vi "CSMP-PostPostMsg.vi"(0 "state":string, 1 "args":string, 2 "source/target":string, 3 "Pre-State in":string, 4 "Pre-Args in":string, 5 "Error in":errorcluster caption="Error in (no error)", 6 "session error":errorcluster, 8 "Module Name":string, 10 "Response Arguments":string) -> (14 "state out":string, 15 "args out":string, 16 "source/target out":string, 17 "Pre-State out":string, 18 "Pre-Args out":string, 19 "error":errorcluster)   [LabVIEW 2020, in "Communicable State Machine.lvlib"]
uses:
  Communicable State Machine.lvlib
  _CSM_MSG_TYPE.ctl
  _Cross CSM State Data.ctl
  _Cross CSM State Response.ctl
  _CSM_Response Source Message.ctl
  Priority Queue.lvclass/Priority Queue.ctl
  Enqueue Element.vi
  _CSMOFGV.vi
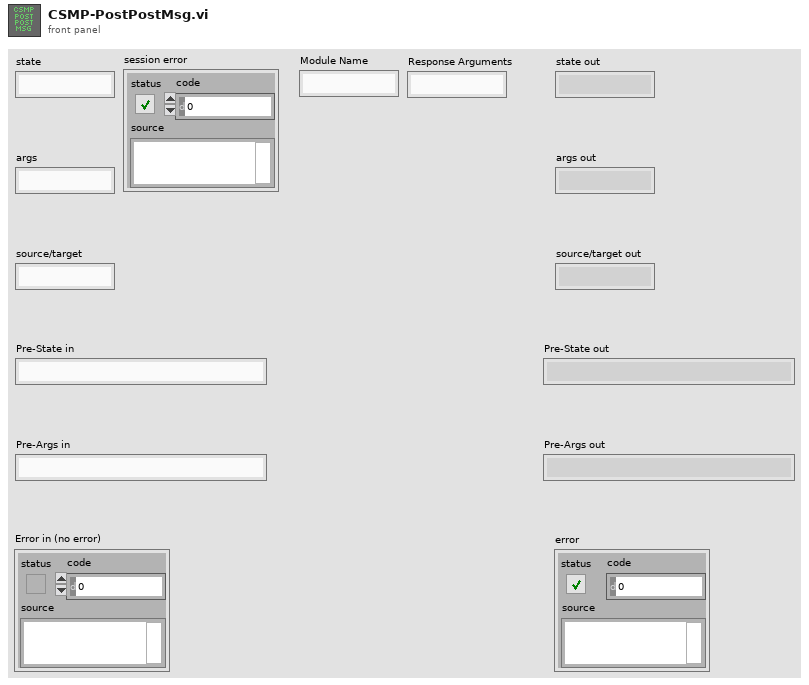
[diagram p1: front panel]
types:
  T1 = typedef "Communicable State Machine.lvlib/_CSMObj.ctl" = cluster{"Requested Name":string, "Module Name":string, "Mode":T2, "Queue":refnum<class "Priority Queue.lvclass">, "CSM-Data":refnum<data-value>, "User Event":refnum<user-event>, "Status Change Event":refnum<user-event>, "Allowed Messages":string[], "Mode-Data":refnum<data-value>, "Group Name":string, "Exit Event":refnum<user-event>}
  T2 = typedef "Communicable State Machine.lvlib/_CSM_MODE.ctl" = enum16{"Not Exist", "Stand Alone", "CSM", "Worker Agent", "Worker", "Chain", "Chain Node"}
  T3 = typedef "Communicable State Machine.lvlib/_CSM_MSG_TYPE.ctl" = enum16{"Sync Message(-@)", "Async Message(->)", "Async without Response(->|)", "Async Response", "Broadcast(-><all>)", "Broadcast(-><status>)", "Broadcast(-><interrupt>)", "Append to JKISM States", "Append to JKISM States(High Priority)"}
  T4 = typedef "Communicable State Machine.lvlib/_Cross CSM State Data.ctl" = cluster{"Msg Type":T3, "state":string, "args":string, "source":string, "RespQ":refnum<queue>, "Response For Message":T5, "Target":string}
  T5 = typedef "Communicable State Machine.lvlib/_CSM_Response Source Message.ctl" = cluster{"‘State":string, "’Arguments":string, "’Error":errorcluster}
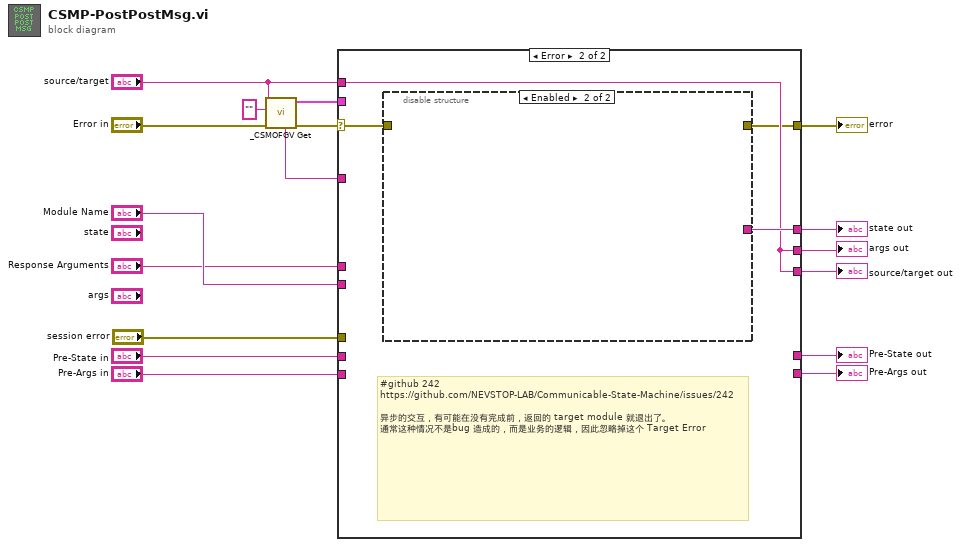
[diagram p0: block diagram]
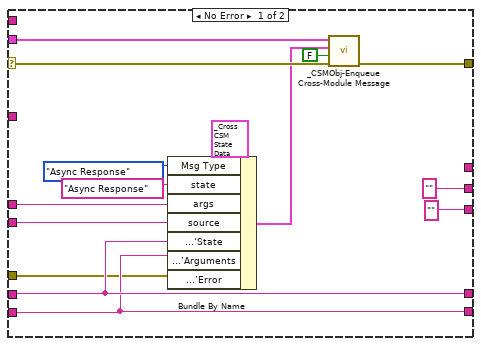
[diagram p2: hidden frame]
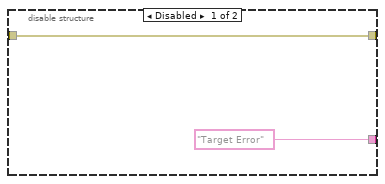
[diagram p3: hidden frame]
diagram:
  n1 = call "_CSMOFGV Get.vi"("Error in"="Error in", "Message"="", "Name(\"\" to use uuid) in"="source/target") -> ("Error out"=w7:errorcluster, "CSM-Obj"=w8:T1, "Name"=w6:string)  [unwired: 6 in]
  n2 = case shown="Error" w7 {
    selector: w7 -> [w31 w33]
    tunnel: w8 -> [w32 _]
    tunnel: [_ w36] -> w5
    tunnel: "source/target" -> [_ w35]
    tunnel: "Response Arguments" -> [w29 _]
    tunnel: "Module Name" -> [w28 _]
    tunnel: w6 -> [_ _]
    tunnel: [w25 _] -> w14
    tunnel: "Pre-State in" -> [w25 _]
    tunnel: "Pre-Args in" -> [w24 _]
    tunnel: [w24 _] -> w13
    tunnel: [w22 w34] -> w16
    tunnel: ["" ("Pre-State out") w35] -> w4
    tunnel: ["" ("Pre-Args out") w35] -> w3
    tunnel: "session error" -> [w18 _]
    frame No Error {
      n3 = Bundle By Name(cluster=T4 {"Msg Type"=enum."Sync Message(-@)", "state"="", "args"="", "source"="", "RespQ"=refnum, "Response For Message"={"‘State"="", "’Arguments"="", "’Error"={"status"=FALSE, "code"=0, "source"=""}}, "Target"=""} ("Cross JKI State Machine State"), "Msg Type"=_CSM_MSG_TYPE."Async Response", "state"="Async Response" ("Response Arguments"), "args"=w29, "source"=w28, "Response For Message.‘State"=w25, "Response For Message.’Arguments"=w24, "Response For Message.’Error"=w18) -> (w27:T4)
      n4 = call "_CSMObj-Enqueue Cross-Module Message.vi"("Error in"=w31, "High Priority?(F)"=FALSE, "Data"=w27, "CSMQ in"=w32) -> ("Error out"=w22:errorcluster)  [unwired: 6 in, 1 out]
    }
    frame Error {
      # "#github 242\nhttps://github.com/NEVSTOP-LAB/Communicable-State-Machine/issues/242\n\n异步的交互，有可能在没有完成前，返回的 target module 就退出了。\n通常这种情况不是bug 造成的，而是业务的逻辑，因此忽略掉这个 Target Error"
      n5 = disable-structure shown="Enabled" {
        disable-tunnel: ["Target Error" ("before match") _] -> w36
        disable-tunnel: [w37 _] -> w34
        disable-tunnel: w33 -> [w37 _]
        frame Disabled {
        }
        frame Enabled {
        }
      }
    }
  }
  "state out" <- w5
  "args out" <- w4
  "source/target out" <- w3
  "error" <- w16
  "Pre-State out" <- w14
  "Pre-Args out" <- w13
